vi "create_client_and_start.vi"(5 "Client type":refnum<class "Client.lvclass">, 8 "error in":errorcluster, 11 "ClientBuilder in":refnum<class "ClientBuilder.lvclass">) -> (0 "error out":errorcluster, 2 "Client out":refnum<class "Client.lvclass">, 3 "ClientBuilder out":refnum<class "ClientBuilder.lvclass">)   [LabVIEW 2020, in "reqwest.lvlib" / "ClientBuilder.lvclass"]
uses:
  ClientBuilder.lvclass
  Client/Client.lvclass
  ClientBuilder.lvclass/ClientBuilder.ctl
  lv_reqwest_64.so
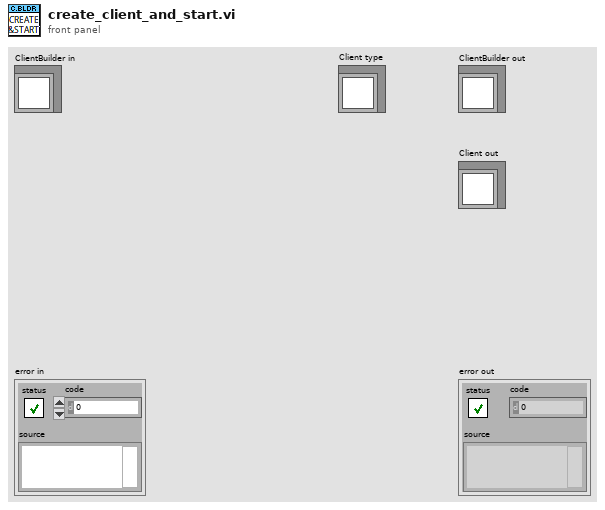
[diagram p1: front panel]
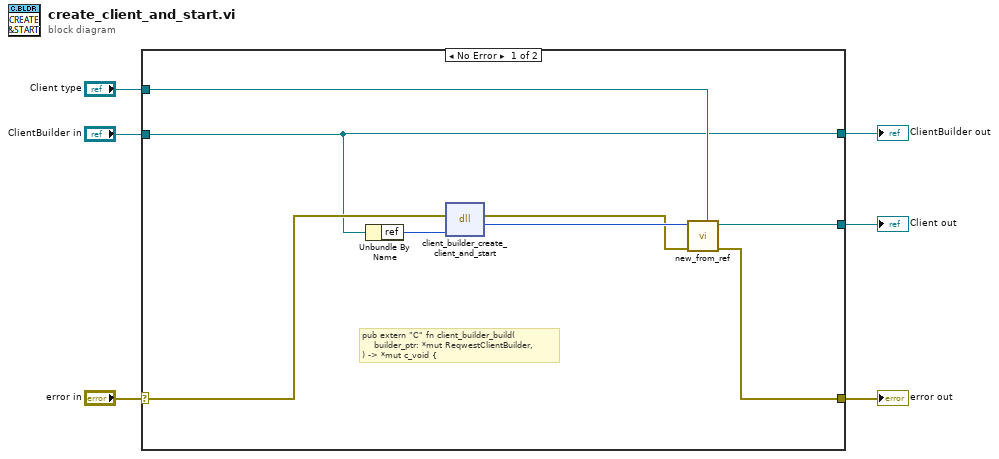
[diagram p0: block diagram]
diagram:
  n1 = case shown="No Error" "error in" {
    selector: "error in" -> [w13 w17]
    tunnel: "ClientBuilder in" -> [w7 w16]
    tunnel: [w9 w17] -> w4
    tunnel: [w11 w15] -> w3
    tunnel: "Client type" -> [w8 w15]
    tunnel: [w7 w16] -> w1
    frame No Error {
      # "pub extern \"C\" fn client_builder_build(\n    builder_ptr: *mut ReqwestClientBuilder,\n) -> *mut c_void {"
      n2 = Unbundle By Name(w7) -> ("ref"=w14:u64)
      n3 = dll-call lib="home/jim-kring/Projects/reqwest-rs-labview/lv_src/lv_reqwest_*.*" fn="client_builder_create_client_and_start"(error in=w13, "client_builder_ref"=w14) -> (error out=w10:errorcluster, "client_ref"=w12:u64)  [unwired: 3 in, 1 out]
      n4 = call "new_from_ref.vi"("Client in"=w8, "error in (no error)"=w10, "client_ref"=w12) -> ("error out"=w9:errorcluster, "Client out"=w11:refnum<class "Client.lvclass">)  [unwired: 7 in]
    }
    frame Error {
    }
  }
  "error out" <- w4
  "Client out" <- w3
  "ClientBuilder out" <- w1
